vi "Is Class Specifier.vi"(11 "Affected Items":T1) -> (3 "Class Specifier Constant?":bool)   [LabVIEW 2023]
doc: "Determine if selected BD object is a class specifier node"
uses:
  top/BundleMagic.ctl
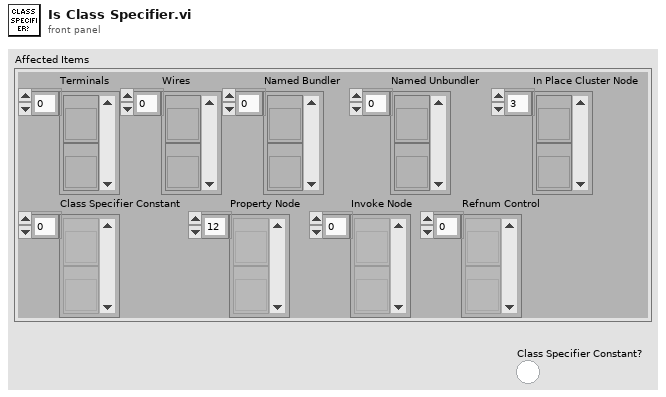
[diagram p1: front panel]
types:
  T1 = typedef "BundleMagic.ctl" = cluster{"Terminals":refnum<vi>[], "Wires":refnum<vi>[], "Named Bundler":refnum<vi>[], "Named Unbundler":refnum<vi>[], "In Place Cluster Node":refnum<vi>[], "Class Specifier Constant":refnum<vi>[], "Property Node":refnum<vi>[], "Invoke Node":refnum<vi>[], "Refnum Control":refnum<vi>[]}
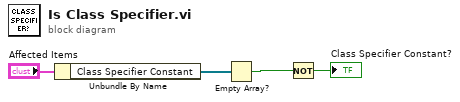
[diagram p0: block diagram]
diagram:
  n1 = Unbundle By Name("Affected Items") -> ("Class Specifier Constant"=w4:refnum<vi>[])
  n2 = Empty Array?(array=w4) -> (empty?=w2:bool)
  n3 = Not(x=w2) -> (.not. x?=→"Class Specifier Constant?":bool)
